vi "2.1.vi"() -> ()   [LabVIEW 2017]
panel:
  out "x*y":i32
  out "dist":i32
  out "depth":i32
  in  "String":string
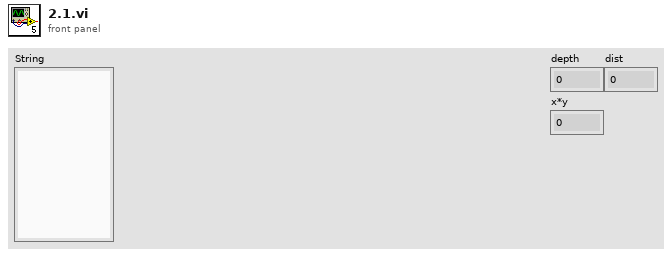
[diagram p1: front panel]
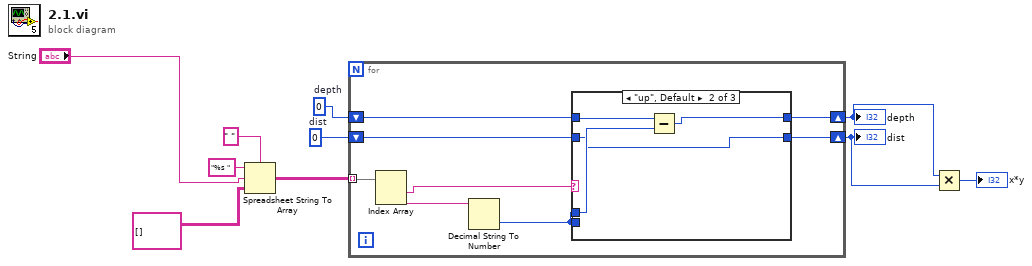
[diagram p0: block diagram]
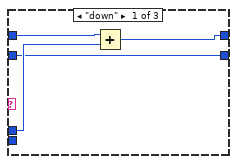
[diagram p2: hidden frame]
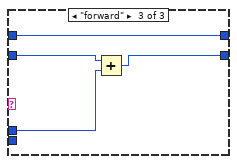
[diagram p3: hidden frame]
diagram:
  w5 = 0  # dist
  w4 = 0  # depth
  n1 = Spreadsheet String To Array(delimiter (Tab)=" ", format string="%s ", spreadsheet string="String", array type (2D Dbl)=string[][] []) -> (array=w6:string[][])
  n2 = for {
    tunnel: w6 -> [w18] mode=indexing
    shift-right: [w13] -> w3
    shift-left: w4 -> [w14]
    shift-right: [w12] -> w2
    shift-left: w5 -> [w15]
    n3 = Index Array(array=w18) -> (element #1=w16:string, element #2=w17:string)  [unwired: 2 in]
    n4 = Decimal String To Number(string=w17) -> (number=w11:i32)  [unwired: 2 in, 1 out]
    n5 = case shown="\"up\", Default" w16 {
      tunnel: w15 -> [w19 w23 w29]
      tunnel: w14 -> [w22 w26 w30]
      tunnel: [w20 w24 w30] -> w13
      tunnel: [w19 w23 w27] -> w12
      tunnel: w11 -> [_ _ _]
      tunnel: w11 -> [w21 w25 w28]
      frame "down" {
        n6 = Add(x=w22, y=w21) -> (x+y=w20:i32)
      }
      frame "up", Default {
        n7 = Subtract(x=w26, y=w25) -> (x-y=w24:i32)
      }
      frame "forward" {
        n8 = Add(x=w29, y=w28) -> (x+y=w27:i32)
      }
    }
  }
  "depth" <- w3
  "dist" <- w2
  n9 = Multiply(x=w3, y=w2) -> (x*y=→"x*y":i32)
